vi "Read Lossless Class.vi"(0 "Depth (Unlimited)":i32=-1, 2 "EnclaveChannel":T1, 3 "error in":errorcluster) -> (7 "Lossless":refnum<class "Lossless.lvclass">, 9 "error out":errorcluster)   [LabVIEW 2022 SP3, in "Enclave.lvlib"]
doc: "Creates a class instance that wraps lossless reads via a queue. As soon as the class is returned it will begin enqueuing data that is written to the Channel Wire or a Writer class instance."
uses:
  Enclave.lvlib
  ))Channel.ctl
  Element.ctl
  Lossless/Lossless.lvclass
  Operation.ctl
  Enclave/Enclave.lvclass
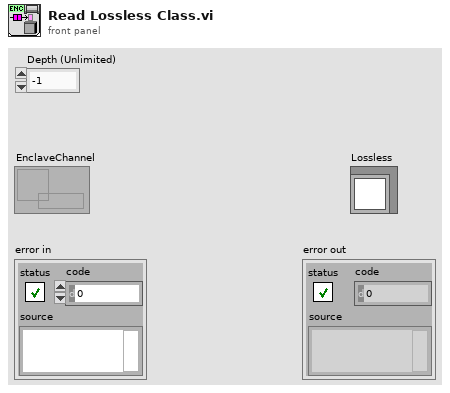
[diagram p1: front panel]
types:
  T1 = typedef "Enclave.lvlib/))Channel.ctl" = refnum<queue>
  T2 = typedef "Enclave.lvlib/Operation.ctl" = enum16{"Get Core", "Init", "Close"}
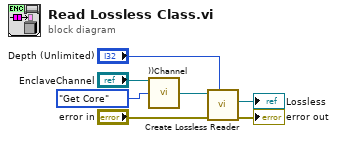
[diagram p0: block diagram]
diagram:
  n1 = call "))Channel.vi"("EnclaveChannel in"="EnclaveChannel", "Operation"=Operation."Get Core") -> ("Enclave"=w5:refnum<class "Enclave.lvclass">)  [unwired: 11 in, 2 out]
  n2 = call "Create Lossless Reader.vi"("Depth (Unlimited)"="Depth (Unlimited)", "error in (no error)"="error in", "Enclave in"=w5) -> ("error out"=→"error out":errorcluster, "Lossless"=→"Lossless":refnum<class "Lossless.lvclass">)  [unwired: 6 in, 1 out]
